vi "auto_ctrl_run_valve_with_pres.vi"(4 "ref_reinit":refnum<vi>, 6 "ref_sp_turn":refnum<vi>, 7 "array_value_in":dbl[](array[numeric]), 9 "sp_in":dbl=49.0 format="%#_13g", 10 "enable_auto_ctrl":bool caption="Auto Control", 11 "ref_fridge_pres":refnum<vi>) -> (0 "status":u32(colorbox)=9567230, 1 "sp_out":dbl format="%.3f", 5 "array_value_out":dbl[](array[numeric]))   [LabVIEW 2019]
doc: "This example demonstrates how to simulate a general PID controller."
uses:
  <vilib>/Analysis/baseanly.llb/Mean (DBL).vi
  <vilib>/addons/control/pid/pid.llb/PID (DBL).vi
  <vilib>/addons/control/pid/NI_PID_pid.lvlib
  <vilib>/Analysis/NI_AALBase.lvlib
panel:
  in  "sp_step":dbl=0.01 format="%.2f"
  in  "sp_nominal":dbl=0.5 format="%.2f"
  in  "sp_max":dbl=2.0 format="%.2f"
  in  "sp_min":dbl=0.3 format="%.2f"
  in  "n_avg":u8=10
  out "MV":dbl format="%.1f"
  in  "P_max":dbl=99.9 format="%.1f"
  in  "P_min":dbl=0.1 format="%.1f"
  out "PID Range":cluster{"High":dbl, "Low":dbl}={"High"=20.0, "Low"=-20.0} {"Low" format="%.1f"; "High" format="%.1f"}
  out "P_in":dbl format="%.1f"
  in  "PID gains":T1={"proportional gain (Kc)"=0.1, "integral time (Ti, min)"=2.0, "derivative time (Td, min)"=0.2} {"derivative time (Td, min)" format="%.4f"; "integral time (Ti, min)" format="%.4f"; "proportional gain (Kc)" format="%.3f"}
  # "Torr"
  # "Torr"
  # "gain = delta_turn / delta_pressure = 0.01 / 0.1 = 0.1"
  # "L/m"
  # "L/m"
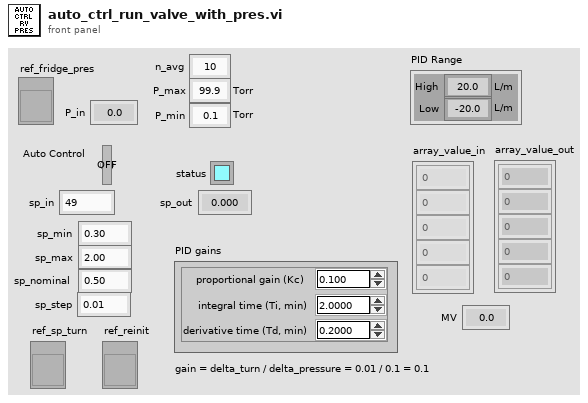
[diagram p1: front panel]
types:
  T1 = cluster{"proportional gain (Kc)":dbl, "integral time (Ti, min)":dbl, "derivative time (Td, min)":dbl}
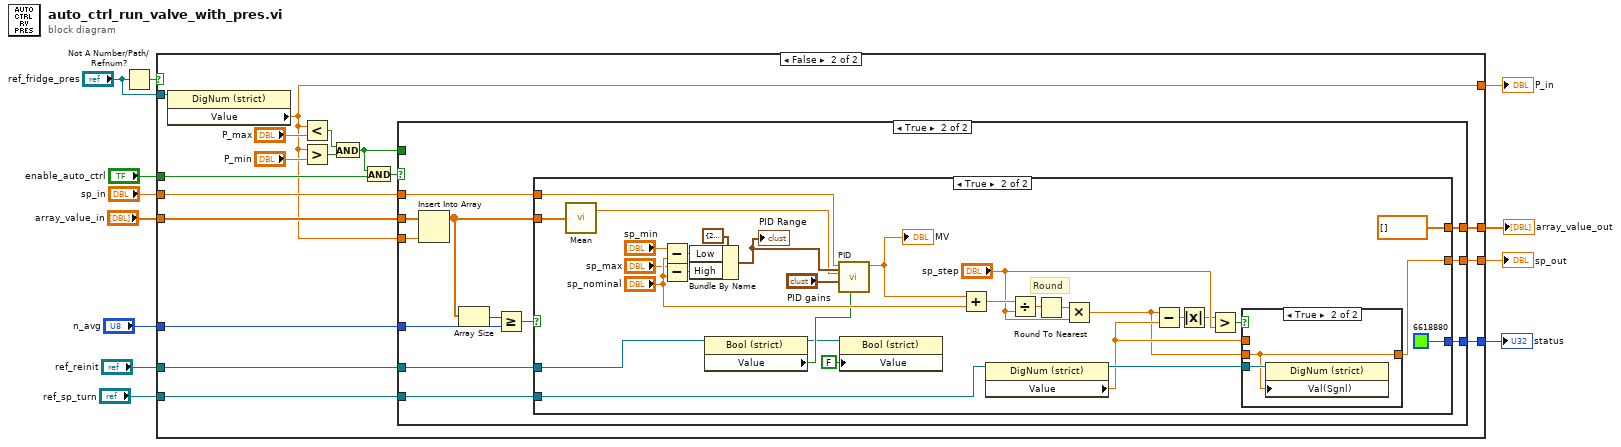
[diagram p0: block diagram]
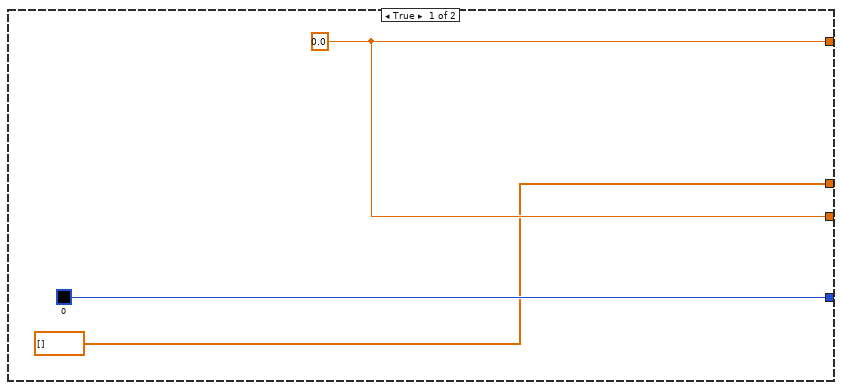
[diagram p2: hidden frame]
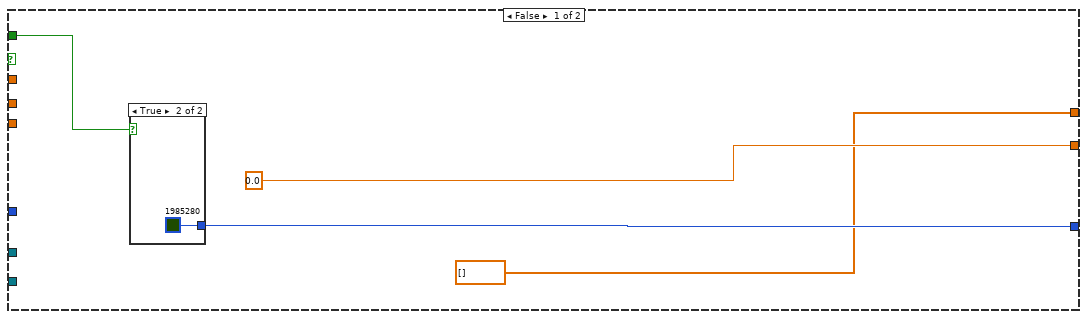
[diagram p3: hidden frame]
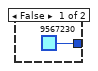
[diagram p4: hidden frame]
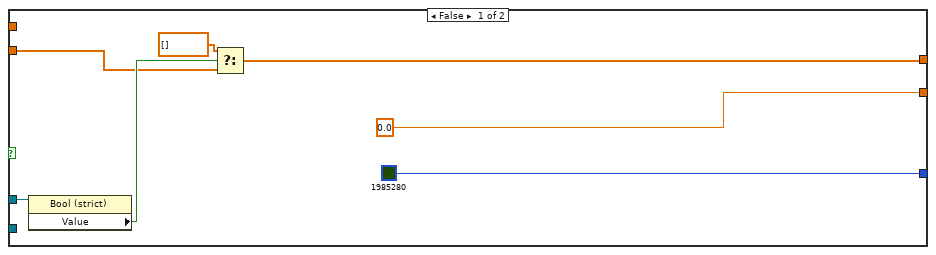
[diagram p5: hidden frame]
diagram:
  n1 = Not A Number/Path/Refnum?(number/path/refnum="ref_fridge_pres") -> (NaN/Path/Refnum?=w8:bool)
  n2 = case shown="False" w8 {
    tunnel: "ref_fridge_pres" -> [_ w30]
    tunnel: [w15 w32] -> w11
    tunnel: [u32 0 ("alarm_status") w31] -> w10
    tunnel: "sp_in" -> [_ w20]
    tunnel: "enable_auto_ctrl" -> [_ w25]
    tunnel: [w15 w16] -> w6
    tunnel: "ref_sp_turn" -> [_ w27]
    tunnel: "ref_reinit" -> [_ w21]
    tunnel: "array_value_in" -> [_ w19]
    tunnel: "n_avg" -> [_ w18]
    tunnel: [dbl[] [] ("f") w17] -> w1
    frame True {
      w15 = 0.0 ("Value")
    }
    frame False {
      n3 = property on="Property Node" class="DigNum (strict)"(reference=w30) -> ("Value"=w16:dbl)  [unwired: 1 in, 2 out]
      n4 = Less?(x=w16, y="P_max") -> (x < y?=w23:bool)
      n5 = Greater?(x=w16, y="P_min") -> (0:w24:bool)
      n6 = And(x=w23, y=w24) -> (x .and. y?=w22:bool)
      n7 = And(x=w22, y=w25) -> (x .and. y?=w26:bool)
      n8 = case shown="True" w26 {
        tunnel: [0.0 ("F_O_new") w48] -> w32
        tunnel: [w34 w50] -> w31
        tunnel: w20 -> [_ w47]
        tunnel: w16 -> [_ w44]
        tunnel: w27 -> [_ w49]
        tunnel: w22 -> [w35 _]
        tunnel: w21 -> [_ w46]
        tunnel: w19 -> [_ w45]
        tunnel: w18 -> [_ w42]
        tunnel: [dbl[] [] ("f") w39] -> w17
        frame False {
          n9 = case shown="True" w35 {
            tunnel: [u32 9567230 ("alarm_status") u32 1985280 ("alarm_status")] -> w34
            frame False {
            }
            frame True {
            }
          }
        }
        frame True {
          n10 = Insert Into Array(array=w45, new element=w44) -> (w40:dbl[])  [unwired: 1 in]
          n11 = Array Size(array=w40) -> (size(s)=w43:i32)
          n12 = Greater Or Equal?(x=w43, y=w42) -> (x >= y?=w41:bool)
          n13 = case shown="True" w41 {
            tunnel: [u32 1985280 ("alarm_status") u32 6618880 ("alarm_status")] -> w50
            tunnel: w49 -> [_ w86]
            tunnel: [0.0 ("F_new") w85] -> w48
            tunnel: w47 -> [_ w83]
            tunnel: w46 -> [w57 w81]
            tunnel: w40 -> [w51 w70]
            tunnel: [w55 dbl[] [] ("f")] -> w39
            frame False {
              n14 = property class="Bool (strict)"(reference=w57) -> ("Value"=w56:bool)  [unwired: 1 in, 2 out]
              n15 = Select(t=dbl[] [] ("f"), s=w56, f=w51) -> (s? t:f=w55:dbl[])
            }
            frame True {
              # "Round"
              n16 = call-poly <vilib>:"Mean.vi"("X"=w70) -> ("mean"=w69:dbl)  [unwired: 1 out]
              n17 = Subtract(x="sp_min", y="sp_nominal") -> (x-y=w75:dbl)
              n18 = Subtract(x="sp_max", y="sp_nominal") -> (x-y=w76:dbl)
              n19 = Bundle By Name(cluster=cluster{"High":dbl, "Low":dbl} {"High"=20.0, "Low"=-20.0} ("PID Range"), "Low"=w75, "High"=w76) -> (w71:cluster{"High":dbl, "Low":dbl})
              "PID Range" <- w71
              n20 = property class="Bool (strict)"(reference=w81) -> (reference out=w79:refnum<vi>, "Value"=w80:bool)  [unwired: 1 in, 1 out]
              n21 = call-poly <vilib>:"PID.vi"("reinitialize? (F)"=w80, "output range"=w71, "PID gains"="PID gains", "process variable"=w69, "setpoint"=w83) -> ("output"=w82:dbl)  [unwired: 5 in, 1 out]
              "MV" <- w82
              n22 = property class="Bool (strict)"(reference=w79, "Value"=FALSE) -> ()  [unwired: 1 in, 2 out]
              n23 = Add(x=w82, y="sp_nominal") -> (x+y=w65:dbl)
              n24 = property class="DigNum (strict)"(reference=w86) -> ("Value"=w67:dbl)  [unwired: 1 in, 2 out]
              n25 = Divide(x=w65, y="sp_step") -> (x/y=w62:dbl)
              n26 = Round To Nearest(number=w62) -> (nearest integer value=w63:dbl)
              n27 = Multiply(x=w63, y="sp_step") -> (x*y=w66:dbl)
              n28 = Subtract(x=w66, y=w67) -> (x-y=w59:dbl)
              n29 = Absolute Value(x=w59) -> (abs(x)=w60:dbl)
              n30 = Greater?(x=w60, y="sp_step") -> (0:w61:bool)
              n31 = case shown="True" w61 {
                tunnel: w86 -> [_ w89]
                tunnel: w66 -> [_ w88]
                tunnel: [w87 w88] -> w85
                tunnel: w67 -> [w87 _]
                frame False {
                }
                frame True {
                  n32 = property class="DigNum (strict)"(reference=w89, "Val(Sgnl)"=w88) -> ()  [unwired: 1 in, 2 out]
                }
              }
            }
          }
        }
      }
    }
  }
  "sp_out" <- w11
  "status" <- w10
  "P_in" <- w6
  "array_value_out" <- w1
